vi "Save Tiff.vi"(5 "Cancelled":bool, 6 "Active Cameras":T3[](array[typedef]), 7 "Stack Info":T1, 8 "error in (no error)":errorcluster, 9 "Frames to Skip":u32, 10 "File Path":path, 11 "Tiff Writer in":refnum<class "Tiff Writer.lvclass">) -> (0 "error out":errorcluster, 3 "Tiff Writer out":refnum<class "Tiff Writer.lvclass">)   [LabVIEW 2023, in "Tiff Writer.lvlib" / "Tiff Writer.lvclass"]
uses:
  Tiff Writer.lvclass
  Resources/Type Defs/Physical Camera Assignment.ctl
  Resources/Type Defs/Stack Info.ctl
  Resources/Type Defs/Camera Type.ctl
  BinaryTIFF/Class/TIFF.lvclass
  Resources/GLOBAL/GLOBAL Time-critical.vi
  Tiff Writer.lvclass/Tiff Writer.ctl
  kernel32.dll
panel:
  in  "Stop Button":bool
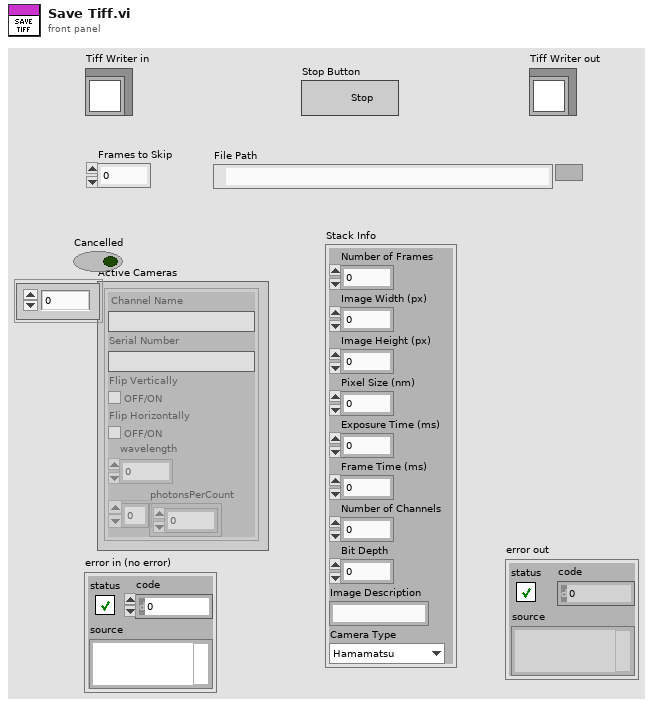
[diagram p1: front panel]
types:
  T1 = typedef "Stack Info.ctl" = cluster{"Number of Frames":u32, "Image Width (px)":u32, "Image Height (px)":u32, "Pixel Size (nm)":dbl, "Exposure Time (ms)":dbl, "Frame Time (ms)":dbl, "Number of Channels":u32, "Bit Depth":u32, "Image Description":string, "Camera Type":T2}
  T2 = typedef "Camera Type.ctl" = enum16{"Hamamatsu", "Andor", "Photometrics"}
  T3 = typedef "Physical Camera Assignment.ctl" = cluster{"Channel Name":string, "Serial Number":string, "Flip Vertically":bool, "Flip Horizontally":bool, "wavelength":i16, "photonsPerCount":dbl[]}
  T4 = cluster{"appended path":path, "Flip Horizontally":bool, "Flip Vertically":bool}[]
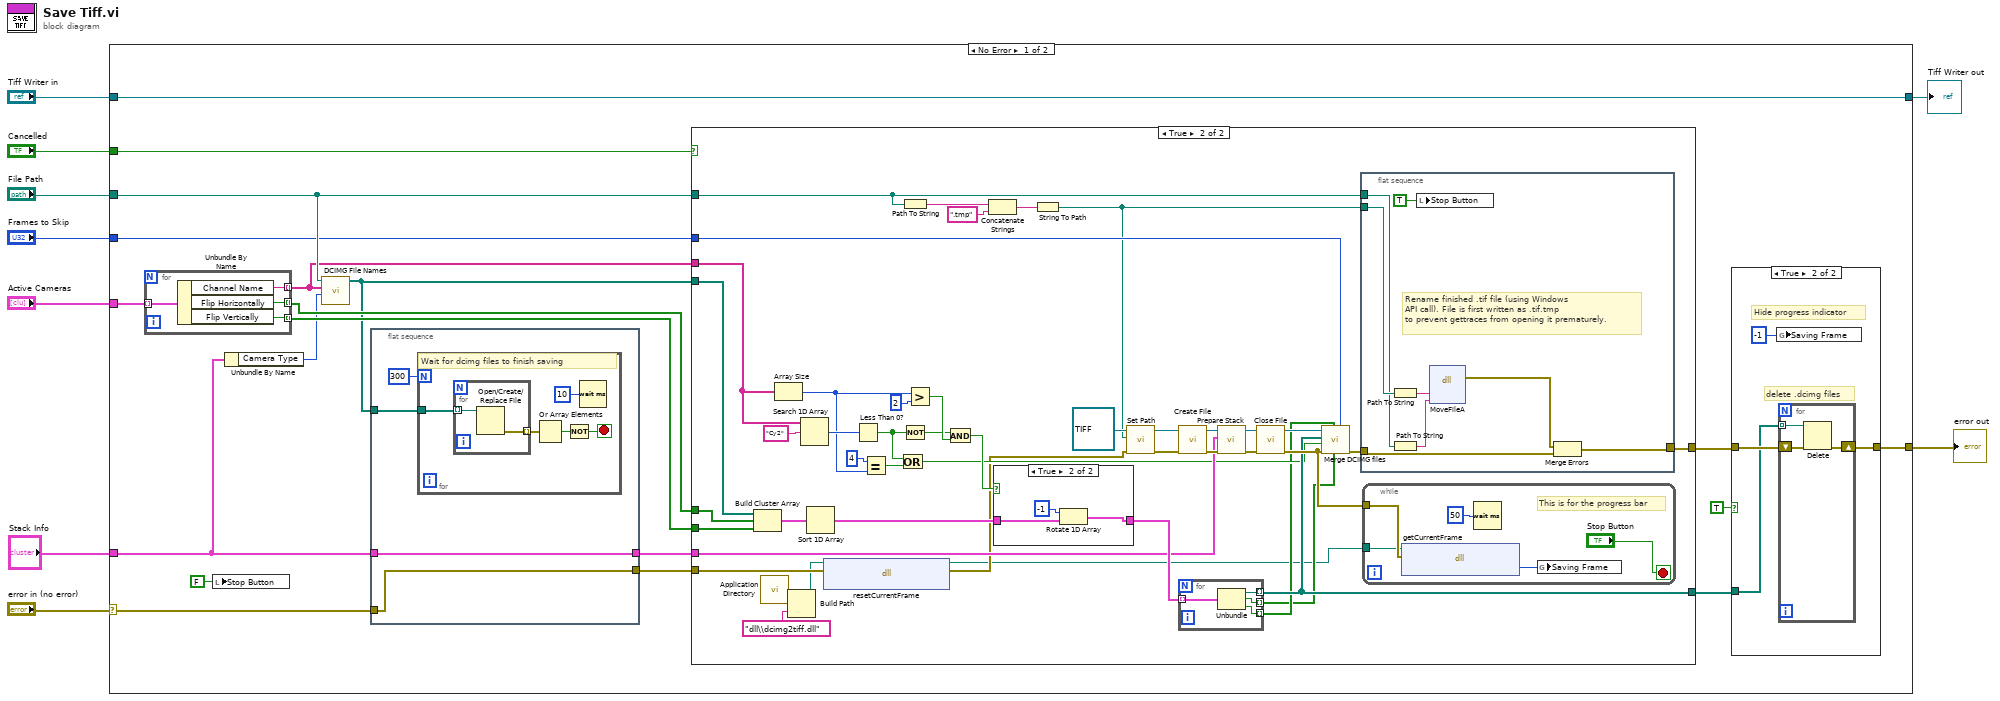
[diagram p0: block diagram]
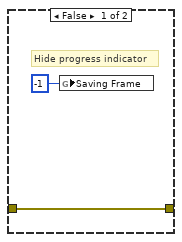
[diagram p4: hidden frame]
diagram:
  n1 = case shown="No Error" "error in (no error)" {
    selector: "error in (no error)" -> [w16 w122]
    tunnel: [w24 w122] -> w8
    tunnel: [w28 w121] -> w6
    tunnel: "Tiff Writer in" -> [w28 w121]
    tunnel: "Stack Info" -> [w11 _]
    tunnel: "File Path" -> [w23 _]
    tunnel: "Active Cameras" -> [w18 _]
    tunnel: "Cancelled" -> [w14 _]
    tunnel: "Frames to Skip" -> [w12 _]
    frame No Error {
      n2 = for {
        tunnel: w18 -> [w43] mode=indexing
        tunnel: [w41] -> w22 mode=indexing
        tunnel: [w42] -> w21 mode=indexing
        tunnel: [w40] -> w20 mode=indexing
        n3 = Unbundle By Name(w43) -> ("Channel Name"=w40:string, "Flip Horizontally"=w41:bool, "Flip Vertically"=w42:bool)
      }
      n4 = local write "Stop Button"(FALSE ("Stop Button")) -> ()
      n5 = Unbundle By Name(w11) -> ("Camera Type"=w10:T2)
      n6 = call "DCIMG File Names.vi"("Camera Type"=w10, "Channel Names"=w20, "TIFF File Path"=w23) -> ("DCIMG Files"=w19:path[])  [unwired: 8 in]
      n7 = flat-sequence {
        tunnel: w19 -> [w32]
        tunnel: w11 -> [w31]
        tunnel: [w31] -> w17
        tunnel: w16 -> [w30]
        tunnel: [w30] -> w15
        frame #0 {
          n8 = for {
            N: 300 -> [_]
            tunnel: w32 -> [w37]
            stop <- w34 stop-if-true
            # "Wait for dcimg files to finish saving"
            n9 = for {
              tunnel: w37 -> [w38] mode=indexing
              tunnel: [w39] -> w36 mode=indexing
              n10 = Open/Create/Replace File(file path (use dialog)=w38) -> (error out=w39:errorcluster)  [unwired: 5 in, 2 out]
            }
            n11 = Or Array Elements(Boolean array=w36) -> (logical OR=w35:bool)
            n12 = Not(x=w35) -> (.not. x?=w34:bool)
            n13 = Wait (ms)(milliseconds to wait=u32 10) -> ()  [unwired: 1 out]
          }
        }
      }
      n14 = case shown="True" w14 {
        tunnel: w23 -> [_ w71]
        tunnel: w15 -> [w44 w54]
        tunnel: w17 -> [_ w63]
        tunnel: [w44 w76] -> w26
        tunnel: [w45 w58] -> w25
        tunnel: w12 -> [_ w59]
        tunnel: w21 -> [_ w78]
        tunnel: w22 -> [_ w77]
        tunnel: w20 -> [_ w51]
        tunnel: w19 -> [w45 w75]
        frame False {
        }
        frame True {
          n15 = Build Cluster Array(w75, w77, w78) -> (w81:T4)
          n16 = call <vilib>:"Application Directory.vi"() -> ("Application Directory"=w48:path)
          n17 = Array Size(array=w51) -> (size(s)=w50:i32)
          n18 = Build Path(base path=w48, name or relative path="dll\\dcimg2tiff.dll") -> (appended path=w47:path)
          n19 = Search 1D Array(1D array=w51, element="Cy2") -> (index of element=w89:i32)  [unwired: 1 in]
          n20 = Sort 1D Array(array=w81) -> (sorted array=w88:T4)
          n21 = dll-call lib="?" fn="resetCurrentFrame"(path in=w47, error in=w54) -> (path out=w46:path, error out=w53:errorcluster)  [unwired: 2 in]
          n22 = Less Than 0?(x=w89) -> (x < 0?=w84:bool)
          n23 = Equal?(x=4, y=w50) -> (x = y?=w83:bool)
          n24 = Or(x=w84, y=w83) -> (x .or. y?=w57:bool)
          n25 = Path To String(path=w71) -> (string=w74:string)
          n26 = Not(x=w84) -> (.not. x?=w79:bool)
          n27 = Greater?(x=w50, y=2) -> (0:w86:bool)
          n28 = And(x=w79, y=w86) -> (x .and. y?=w85:bool)
          n29 = Concatenate Strings(w74, ".tmp" ("string")) -> (w72:string)
          n30 = case shown="True" w85 {
            tunnel: w88 -> [w95 w98]
            tunnel: [w95 w97] -> w80
            frame False {
            }
            frame True {
              n31 = Rotate 1D Array(1:w98, 2:-1 ("n")) -> (0:w97:T4)
            }
          }
          n32 = String To Path(string=w72) -> (path=w52:path)
          n33 = call-dynamic "Set Path.vi"("error in (no error)"=w53, "File Path"=w52, "TIFF in"=refnum<class "TIFF.lvclass"> refnum ("BinaryTIFF.lvlib:TIFF.lvclass")) -> ("error out"=w70:errorcluster, "TIFF out"=w66:refnum<class "TIFF.lvclass">)  [unwired: 7 in]
          n34 = call-dynamic "Create File.vi"("error in (no error)"=w70, "TIFF in"=w66) -> ("error out"=w69:errorcluster, "TIFF out"=w65:refnum<class "TIFF.lvclass">)  [unwired: 8 in]
          n35 = for {
            tunnel: w80 -> [w94] mode=indexing
            tunnel: [w93] -> w58 mode=indexing
            tunnel: [w92] -> w55 mode=indexing
            tunnel: [w91] -> w56 mode=indexing
            n36 = Unbundle(w94) -> ("appended path"=w93:path, "Flip Horizontally"=w92:bool, "Flip Vertically"=w91:bool)
          }
          n37 = call-dynamic "Prepare Stack.vi"("error in (no error)"=w69, "Stack Info"=w63, "TIFF in"=w65) -> ("error out"=w68:errorcluster, "TIFF out"=w64:refnum<class "TIFF.lvclass">)  [unwired: 7 in]
          n38 = call-dynamic "Close File.vi"("error in (no error)"=w68, "TIFF in"=w64) -> ("error out"=w61:errorcluster, "TIFF out"=w62:refnum<class "TIFF.lvclass">)  [unwired: 8 in]
          n39 = call-dynamic "Merge DCIMG files.vi"("Frames to Skip"=w59, "Horizontal Flip"=w55, "Vertical Flip"=w56, "error in (no error)"=w61, "Channel 3 Right?"=w57, "DCIMG Paths (2 to 4)"=w58, "TIFF in"=w62) -> ("error out"=w60:errorcluster)  [unwired: 3 in, 1 out]
          n40 = flat-sequence {
            tunnel: w60 -> [w102]
            tunnel: w52 -> [w104]
            tunnel: w71 -> [w99]
            tunnel: [w101] -> w76
            frame #0 {
              # "Rename finished .tif file (using Windows\nAPI call). File is first written as .tif.tmp\nto prevent gettraces from opening it prematurely."
              n41 = Path To String(path=w104) -> (string=w105:string)
              n42 = Path To String(path=w99) -> (string=w100:string)
              n43 = local write "Stop Button"(TRUE ("Stop Button")) -> ()
              n44 = dll-call lib="kernel32.dll" fn="MoveFileA"("arg1"=w105, "arg2"=w100) -> (error out=w103:errorcluster)  [unwired: 6 in, 1 out]
              n45 = Merge Errors(w103, w102) -> (w101:errorcluster)
            }
          }
          n46 = while {
            tunnel: w61 -> [w109]
            tunnel: w46 -> [w107]
            stop <- "Stop Button" stop-if-true
            # "This is for the progress bar"
            n47 = dll-call lib="?" fn="getCurrentFrame"(path in=w107, error in=w109) -> ("Current Frame"=w108:u64)  [unwired: 1 in, 2 out]
            n48 = Wait (ms)(milliseconds to wait=u32 50) -> ()  [unwired: 1 out]
            n49 = global write "GLOBAL Time-critical.vi" "Saving Frame"(w108) -> ()
          }
        }
      }
      n50 = case shown="True" TRUE {
        tunnel: [w113 w117] -> w24
        tunnel: w26 -> [w113 w116]
        tunnel: w25 -> [_ w115]
        frame False {
          # "Hide progress indicator"
          n51 = global write "GLOBAL Time-critical.vi" "Saving Frame"(-1 ("Saving Frame")) -> ()
        }
        frame True {
          # "Hide progress indicator"
          # "delete .dcimg files"
          n52 = global write "GLOBAL Time-critical.vi" "Saving Frame"(-1 ("Saving Frame")) -> ()
          n53 = for {
            shift-right: [w118] -> w117
            shift-left: w116 -> [w119]
            tunnel: w115 -> [w120] mode=indexing
            n54 = Delete(path (use dialog)=w120, error in=w119) -> (error out=w118:errorcluster)  [unwired: 3 in, 2 out]
          }
        }
      }
    }
    frame Error {
    }
  }
  "error out" <- w8
  "Tiff Writer out" <- w6
